vi "Close TDMS.vi"(8 "error in (no error)":errorcluster, 11 "Sparkfun Atomic IMU in":refnum<class "Sparkfun Atomic IMU.lvclass">) -> (0 "error out":errorcluster, 3 "Sparkfun Atomic IMU out":refnum<class "Sparkfun Atomic IMU.lvclass">)   [LabVIEW 2019, in "Sparkfun Atomic IMU.lvclass"]
doc: "Closes the tdms file."
uses:
  Sparkfun Atomic IMU.lvclass
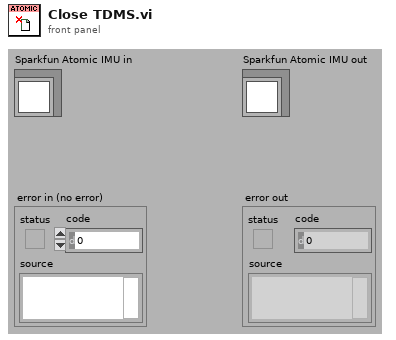
[diagram p1: front panel]
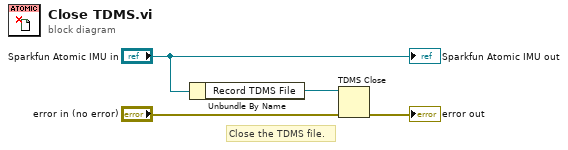
[diagram p0: block diagram]
diagram:
  # "Close the TDMS file."
  n1 = Unbundle By Name("Sparkfun Atomic IMU in") -> ("Record TDMS File"=w3:refnum<k34>)
  n2 = TDMS Close(8:"error in (no error)", 11:w3) -> (0:→"error out":errorcluster)  [unwired: 1 out]
  "Sparkfun Atomic IMU out" <- "Sparkfun Atomic IMU in"
